vi "Configure.vi"(8 "error in (no error)":errorcluster, 11 "Mag Lab Measure Controller in":refnum<class "Mag Lab Measure Controller.lvclass">) -> (0 "error out":errorcluster, 3 "Mag Lab Measure Controller out":refnum<class "Mag Lab Measure Controller.lvclass">)   [LabVIEW 2015, in "Mag Lab Measure Controller.lvclass"]
uses:
  Mag Lab Measure Controller.lvclass
  Mag Lab Error Handler/Mag Lab Error Handler.lvclass
  Mag Lab Measure Base/Mag Lab Measure Base.lvclass/Mag Lab Measure Base.ctl
  Mag Lab Error Handler/Mag Lab Error Handler.lvclass/Mag Lab Error Handler.ctl
  Mag Lab Measure Controller.lvclass/Mag Lab Measure Controller.ctl
  Compound Measurement/Compound Measurement.lvclass
  Mag Lab Measure Base/Mag Lab Measure Base.lvclass
  <vilib>/ActorFramework/Actor/Actor.lvclass
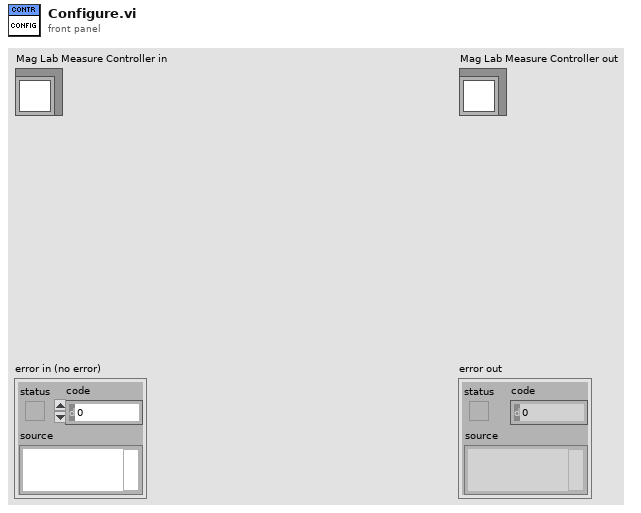
[diagram p1: front panel]
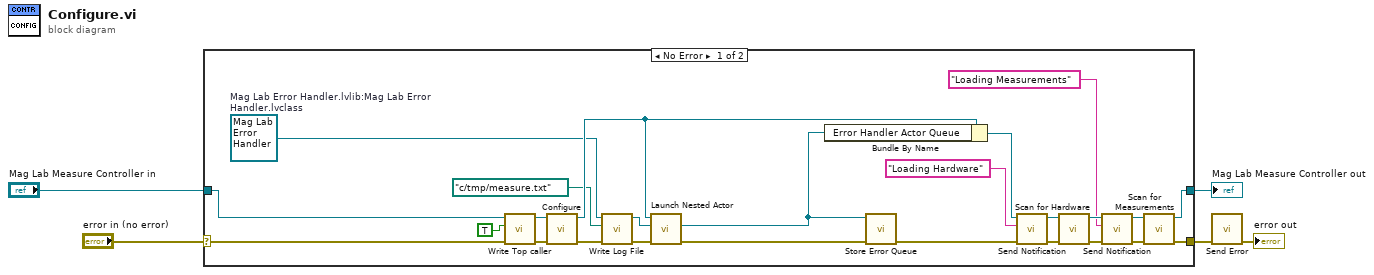
[diagram p0: block diagram]
diagram:
  n1 = case shown="No Error" "error in (no error)" {
    selector: "error in (no error)" -> [w25 w31]
    tunnel: [w27 w31] -> w2
    tunnel: "Mag Lab Measure Controller in" -> [w24 w32]
    tunnel: [w28 w32] -> w3
    frame No Error {
      w10 = refnum<class "Mag Lab Error Handler.lvclass"> refnum  # Mag Lab Error Handler.lvlib:Mag Lab Error Handler.lvclass
      n2 = call "Write Top caller.vi"("error in (no error)"=w25, "Top caller"=TRUE, "Mag Lab Measure Base in"=w24) -> ("error out"=w26:errorcluster, "Mag Lab Measure Base out"=w23:refnum<class "Mag Lab Measure Controller.lvclass">)  [unwired: 7 in]
      n3 = call-parent "Configure.vi"("error in (no error)"=w26, "Mag Lab Root in"=w23) -> ("error out"=w8:errorcluster, "Mag Lab Root out"=w21:refnum<class "Mag Lab Measure Controller.lvclass">)  [unwired: 8 in]
      n4 = call "Write Log File.vi"("error in (no error)"=w8, "Log File"=path "c:/tmp/measure.txt", "Mag Lab Error Handler in"=w10) -> ("error out"=w7:errorcluster, "Mag Lab Error Handler out"=w9:refnum<class "Mag Lab Error Handler.lvclass">)  [unwired: 7 in]
      n5 = call <vilib>:"Launch Nested Actor.vi"("error in (no error)"=w7, "Nested Actor"=w9, "Caller Actor in"=w21) -> ("error out"=w30:errorcluster, "Nested Actor's Enqueuer"=w29:refnum<class "Message Enqueuer.lvclass">)  [unwired: 6 in, 1 out]
      n6 = Bundle By Name(cluster=w21, "Error Handler Actor Queue"=w29) -> (w18:refnum<class "Mag Lab Measure Controller.lvclass">)
      n7 = call "Store Error Queue.vi"("error in (no error)"=w30, "Error Handler Queue"=w29) -> ("error out"=w17:errorcluster)  [unwired: 9 in]
      n8 = call-dynamic "Send Notification.vi"("error in (no error)"=w17, "Notification"="Loading Hardware" ("Message"), "Mag Lab Measure Controller in"=w18) -> ("error out"=w19:errorcluster, "Mag Lab Measure Controller out"=w16:refnum<class "Mag Lab Measure Controller.lvclass">)  [unwired: 7 in]
      n9 = call-dynamic "Scan for Hardware.vi"("error in (no error)"=w19, "Mag Lab Measure Controller in"=w16) -> ("error out"=w11:errorcluster, "Mag Lab Measure Controller out"=w15:refnum<class "Mag Lab Measure Controller.lvclass">)  [unwired: 8 in]
      n10 = call-dynamic "Send Notification.vi"("error in (no error)"=w11, "Notification"="Loading Measurements" ("Message"), "Mag Lab Measure Controller in"=w15) -> ("error out"=w13:errorcluster, "Mag Lab Measure Controller out"=w14:refnum<class "Mag Lab Measure Controller.lvclass">)  [unwired: 7 in]
      n11 = call-dynamic "Scan for Measurements.vi"("error in (no error)"=w13, "Mag Lab Measure Controller in"=w14) -> ("error out"=w27:errorcluster, "Mag Lab Measure Controller out"=w28:refnum<class "Mag Lab Measure Controller.lvclass">)  [unwired: 8 in]
    }
    frame Error {
    }
  }
  "Mag Lab Measure Controller out" <- w3
  n12 = call "Send Error.vi"("error in (no error)"=w2) -> ("error out"=→"error out":errorcluster)  [unwired: 9 in, 1 out]
